vi "Initialize.vi"(8 "error in (no error)":errorcluster, 9 "Camera Type":T1, 10 "DAQ Configuration":T2={"Shutters"=[], "fluidics trigger line"="Dev1/port1/line1", "camera trigger line"="", "COM Port"="COM5", "Device type"=enum."Microsync"}, 11 "Synchronization Device in":refnum<class "Microsync.lvclass">) -> (0 "error out":errorcluster, 3 "Synchronization Device out":refnum<class "Microsync.lvclass">, 4 "Trigger Jitter (ms)":dbl)   [LabVIEW 2023, in "Microsync.lvlib" / "Microsync.lvclass"]
uses:
  Microsync.lvclass
  Resources/Type Defs/DAQ Configuration.ctl
  Resources/Type Defs/Shutter Configuration.ctl
  Resources/Type Defs/Sync Device Type.ctl
  Resources/Type Defs/Camera Type.ctl
  <vilib>/Instr/_visa.llb/VISA Flush IO Buffer Mask.ctl
  Microsync.lvclass/Microsync.ctl
  <vilib>/Instr/_visa.llb/VISA Configure Serial Port (Instr).vi
panel:
  in  "Shutter delay, us":u32=1900
  in  "Required firmware version":string="2.4."
  out "Detected firmware version":string
  out "Startup message":string
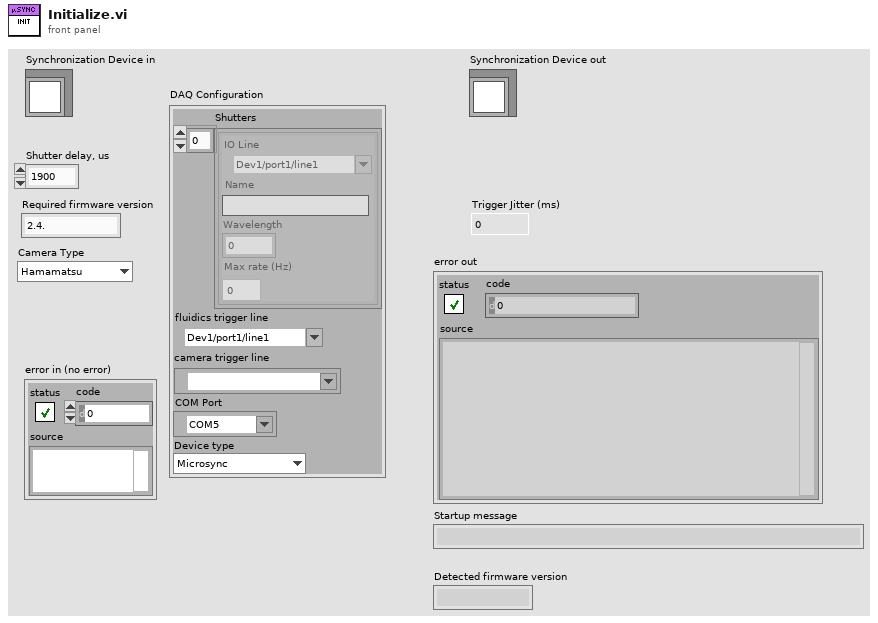
[diagram p1: front panel]
types:
  T1 = typedef "Camera Type.ctl" = enum16{"Hamamatsu", "Andor", "Photometrics"}
  T2 = typedef "DAQ Configuration.ctl" = cluster{"Shutters":T3[], "fluidics trigger line":tag, "camera trigger line":tag, "COM Port":refnum<visa-resource-name>, "Device type":T4}
  T3 = typedef "Shutter Configuration.ctl" = cluster{"IO Line":tag, "Name":string, "Wavelength":u16, "Max rate (Hz)":dbl}
  T4 = typedef "Sync Device Type.ctl" = enum16{"Disabled", "NI DAQ", "Arduino DAQ", "Microsync"}
  T5 = enum16{"ro_VERSION", "ro_SYS_TIMER_STATUS", "ro_SYS_TIMER_VALUE", "ro_SYS_TIMER_OVF_COUNT", "ro_SYS_TIME_ms", "ro_SYS_TIMER_PRESCALER", "rw_DFLT_PULSE_DURATION_us", "ro_WATCHDOG_TIMEOUT_ms", "ro_N_EVENTS", "rw_INTLCK_ENABLED", "rw_SELECTED_LASERS", "wo_OPEN_SHUTTERS", "wo_CLOSE_SHUTTERS", "rw_SHUTTER_DELAY_us", "rw_CAM_READOUT_us", "rw_CAM_GLOBAL_RST"}
  T6 = typedef "VISA Flush IO Buffer Mask.ctl" = u16
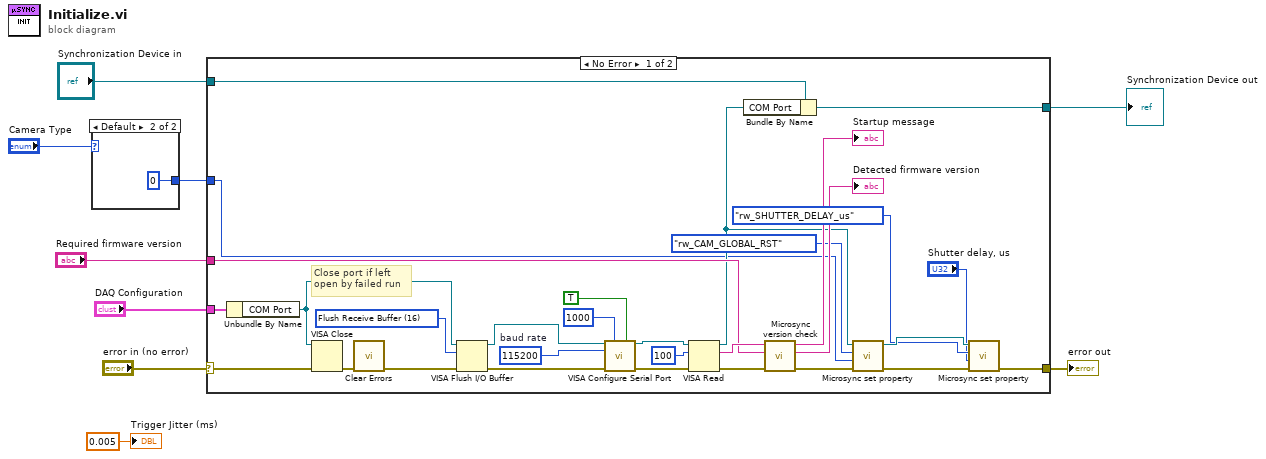
[diagram p0: block diagram]
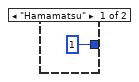
[diagram p2: hidden frame]
diagram:
  n1 = case shown="Default" "Camera Type" {
    tunnel: [u32 1 ("Property value") u32 0 ("Property value")] -> w1
    frame "Hamamatsu" {
    }
    frame Default {
    }
  }
  n2 = case shown="No Error" "error in (no error)" {
    selector: "error in (no error)" -> [w38 w42]
    tunnel: [w28 w43] -> w8
    tunnel: "Synchronization Device in" -> [w29 w43]
    tunnel: [w15 w42] -> w6
    tunnel: "DAQ Configuration" -> [w41 _]
    tunnel: "Required firmware version" -> [w32 _]
    tunnel: w1 -> [w17 _]
    frame No Error {
      w23 = T6 16 items=["Flush Receive Buffer"=16, "Write Transmit Buffer to Device"=32, "Flush Receive Buffer (No I/O)"=64, "Flush Transmit Buffer"=128] ("Mask")
      w37 = u32 115200  # baud rate
      # "Close port if left\nopen by failed run"
      n3 = Unbundle By Name(w41) -> ("COM Port"=w26:refnum<visa-resource-name>)
      n4 = VISA Close(VISA resource name=w26, error in (no error)=w38) -> (error out=w39:errorcluster)
      n5 = call <vilib>:"Clear Errors.vi"("error in (no error)"=w39) -> ("error out"=w27:errorcluster)  [unwired: 5 in, 1 out]
      n6 = VISA Flush I/O Buffer(VISA resource name=w26, mask (16)=w23, error in (no error)=w27) -> (VISA resource name out=w25:refnum<visa-resource-name>, error out=w24:errorcluster)
      n7 = call-poly "VISA Configure Serial Port"("VISA resource name"=w25, "timeout (10sec)"=u32 1000, "Enable Termination\nChar (T)"=TRUE ("Enable Termination\nChar (T)"), "baud rate (9600)"=w37, "error in (no error)"=w24) -> ("VISA resource name out"=w35:refnum<visa-resource-name>, "error out"=w40:errorcluster)  [unwired: 9 in]
      n8 = VISA Read(VISA resource name=w35, byte count=u32 100, error in (no error)=w40) -> (VISA resource name out=w19:refnum<visa-resource-name>, read buffer=w33:string, error out=w34:errorcluster)  [unwired: 1 out]
      n9 = Bundle By Name(cluster=w29, "COM Port"=w19) -> (w28:refnum<class "Microsync.lvclass">)
      n10 = call "Microsync version check.vi"("error in (no error)"=w34, "Required firmware version"=w32, "Startup message"=w33) -> ("error out"=w20:errorcluster, "Detected firmware version"=→"Detected firmware version":string, "Startup message"=→"Startup message":string)  [unwired: 6 in]
      n11 = call "Microsync set property.vi"("error in (no error)"=w20, "Property value"=w17, "property to set"=T5."rw_CAM_GLOBAL_RST", "VISA resource name"=w19) -> ("error out"=w16:errorcluster, "VISA resource name out"=w14:refnum<visa-resource-name>)  [unwired: 6 in]
      n12 = call "Microsync set property.vi"("error in (no error)"=w16, "Property value"="Shutter delay, us", "property to set"=T5."rw_SHUTTER_DELAY_us", "VISA resource name"=w14) -> ("error out"=w15:errorcluster)  [unwired: 6 in, 1 out]
    }
    frame Error {
    }
  }
  "error out" <- w6
  "Synchronization Device out" <- w8
  "Trigger Jitter (ms)" <- 0.005 ("Trigger Jitter (ms)")
